vi "Lesson 1-1 Getting started with myDAQ.vi"() -> ()   [LabVIEW 2020]
uses:
  <vilib>/DAQmx/read.llb/DAQmx Read (Analog 1D DBL 1Chan NSamp).vi
  <vilib>/DAQmx/create/channels.llb/DAQmx Create Channel (AI-Voltage-Basic).vi
  <vilib>/DAQmx/configure/timing.llb/DAQmx Timing (Sample Clock).vi
  <vilib>/DAQmx/miscellaneous.llb/DAQmx Fill In Error Info.vi
panel:
  out "error out":errorcluster
  in  "stop":bool
  out "Waveform Chart":dbl[](graph)
  out "data":dbl[](array[numeric]) format="%0.2f"
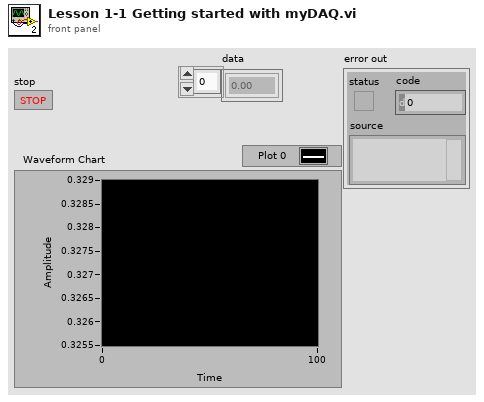
[diagram p1: front panel]
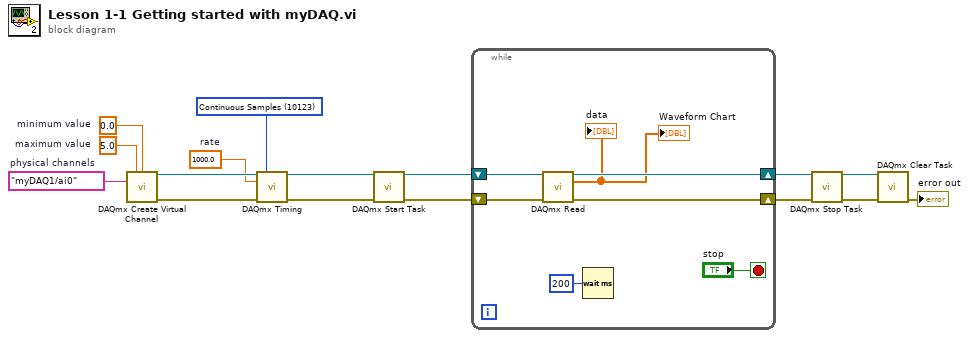
[diagram p0: block diagram]
diagram:
  w2 = 1000.0  # rate
  w3 = 10123 items=["Finite Samples"=10178, "Continuous Samples"=10123, "Hardware Timed Single Point"=12522] ("sample mode")
  w4 = tag "myDAQ1/ai0"  # physical channels
  w5 = 0.0  # minimum value
  w6 = 5.0  # maximum value
  n1 = call-poly <vilib>:"DAQmx Create Virtual Channel.vi"("maximum value"=w6, "minimum value"=w5, "physical channels"=w4) -> ("task out"=w16:refnum<k21>, "error out"=w15:errorcluster)  [unwired: 11 in]
  n2 = call-poly <vilib>:"DAQmx Timing.vi"("task/channels in"=w16, "sample mode"=w3, "rate"=w2, "error in"=w15) -> ("task out"=w14:refnum<k21>, "error out"=w13:errorcluster)  [unwired: 10 in]
  n3 = call <vilib>:"DAQmx Start Task.vi"("task/channels in"=w14, "error in"=w13) -> ("task out"=w12:refnum<k21>, "error out"=w11:errorcluster)  [unwired: 12 in]
  n4 = while {
    shift-right: [w21] -> w10
    shift-left: w12 -> [w23]
    shift-right: [w20] -> w9
    shift-left: w11 -> [w22]
    stop <- "stop" stop-if-true
    n5 = call-poly <vilib>:"DAQmx Read.vi"("task/channels in"=w23, "error in"=w22) -> ("task out"=w21:refnum<k21>, "data"=→"data" →"Waveform Chart":dbl[], "error out"=w20:errorcluster)  [unwired: 11 in]
    n6 = Wait (ms)(milliseconds to wait=u32 200) -> ()  [unwired: 1 out]
  }
  n7 = call <vilib>:"DAQmx Stop Task.vi"("task/channels in"=w10, "error in"=w9) -> ("task out"=w8:refnum<k21>, "error out"=w7:errorcluster)  [unwired: 12 in]
  n8 = call <vilib>:"DAQmx Clear Task.vi"("task in"=w8, "error in"=w7) -> ("error out"=→"error out":errorcluster)  [unwired: 13 in]
